vi "Create.vi"(8 "error in (no error)":errorcluster, 10 "Suite Name":string) -> (0 "error out":errorcluster, 3 "LUnit Test Suite V2 out":refnum<class "LUnit Test Suite V2.lvclass">)   [LabVIEW 2020, in "LUnit Test Suite V2.lvclass"]
uses:
  LUnit Test Suite V2.lvclass
  LUnit Test Suite V2.lvclass/LUnit Test Suite V2.ctl
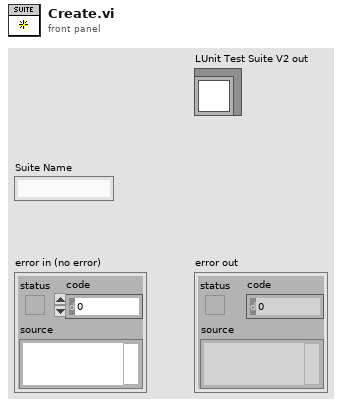
[diagram p1: front panel]
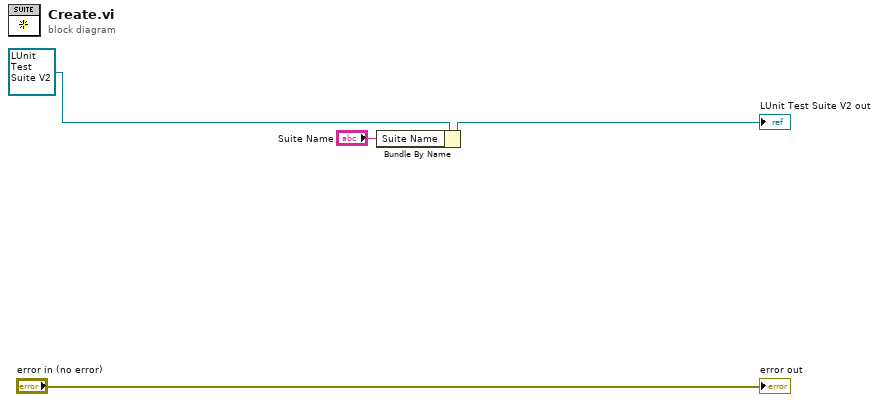
[diagram p0: block diagram]
diagram:
  n1 = Bundle By Name(cluster=refnum<class "LUnit Test Suite V2.lvclass"> refnum ("LUnit Test Suite V2 in"), "Suite Name"="Suite Name") -> (→"LUnit Test Suite V2 out":refnum<class "LUnit Test Suite V2.lvclass">)
  "error out" <- "error in (no error)"
